vi "Parse JSON for Channels.vi"(8 "error in":errorcluster, 11 "JSON":string) -> (0 "error out":errorcluster, 2 "Channel JSON List":string[](array[string]), 3 "Channel Type List":string[](array[string]))   [LabVIEW 2026, in "Template Deployment Hooks.lvlib"]
uses:
  Template Deployment Hooks.lvlib
  <vilib>/regexp/Match Regular Expression.xnode
  <vilib>/JDP Science/JSONtext/JSONtext.lvlib
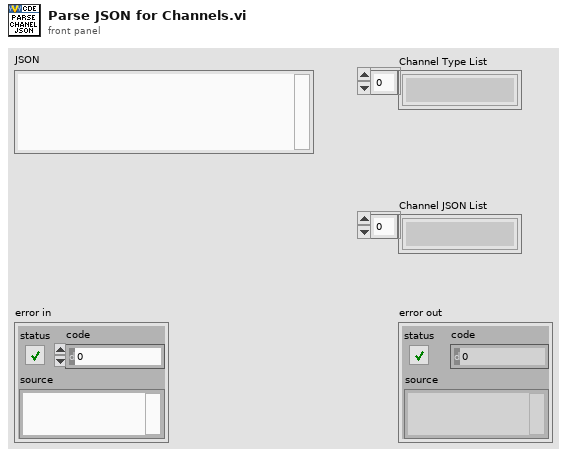
[diagram p1: front panel]
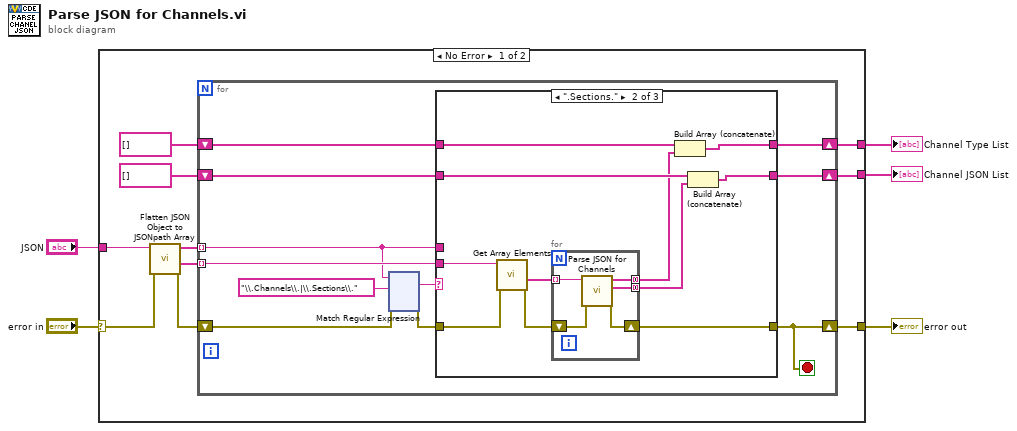
[diagram p0: block diagram]
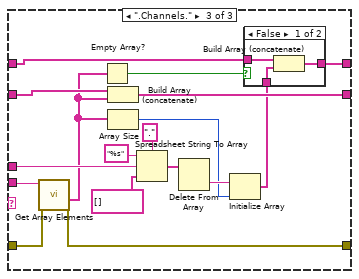
[diagram p3: hidden frame]
diagram:
  n1 = case shown="No Error" "error in" {
    selector: "error in" -> [w14 w184]
    tunnel: [w13 w184] -> w5
    tunnel: "JSON" -> [w9 _]
    tunnel: [w7 _] -> w2
    tunnel: [w6 _] -> w1
    frame No Error {
      n2 = call <vilib>:"Flatten JSON Object to JSONpath Array.vi"("error in (no error)"=w14, "JSON"=w9) -> ("error out"=w15:errorcluster, "<JSON>"=w11:string[], "$Paths"=w12:string[])  [unwired: 7 in]
      n3 = for {
        tunnel: w12 -> [w18] mode=indexing
        shift-right: [w22] -> w6
        shift-left: string[] [] ("<JSON>") -> [w23]
        tunnel: w11 -> [w21] mode=indexing
        shift-right: [w26] -> w13
        shift-left: w15 -> [w25]
        shift-right: [w19] -> w7
        shift-left: string[] [] -> [w20]
        stop <- w26 stop-if-true
        n4 = xnode "Match Regular Expression"("input string"=w18, "regular expression"="\\.Channels\\.|\\.Sections\\.", "error in"=w25) -> ("whole match"=w16:string, "error out"=w24:errorcluster)  [unwired: 3 in, 3 out]
        n5 = case shown="\".Sections.\"" w16 {
          tunnel: [w29 w38 w61] -> w26
          tunnel: w23 -> [w27 w37 w60]
          tunnel: [w27 w31 w59] -> w22
          tunnel: w21 -> [_ w36 w51]
          tunnel: w20 -> [w28 w35 w52]
          tunnel: [w28 w33 w53] -> w19
          tunnel: w24 -> [w29 w40 w62]
          tunnel: w18 -> [_ _ w54]
          frame Default {
          }
          frame ".Sections." {
            n6 = call <vilib>:"Get Array Elements.vi"("error in (no error)"=w40, "JSON"=w36) -> ("error out"=w39:errorcluster, "<JSON>"=w34:string[])  [unwired: 7 in, 1 out]
            n7 = for {
              tunnel: w34 -> [w43] mode=indexing
              tunnel: [w42] -> w32 mode=concatenating
              tunnel: [w41] -> w30 mode=concatenating
              shift-right: [w44] -> w38
              shift-left: w39 -> [w45]
              n8 = call "Parse JSON for Channels.vi"("error in"=w45, "JSON"=w43) -> ("error out"=w44:errorcluster, "Channel JSON List"=w41:string[], "Channel Type List"=w42:string[])  [unwired: 7 in]
            }
            n9 = Build Array (concatenate)(w35, w32) -> (w33:string[])
            n10 = Build Array (concatenate)(w37, w30) -> (w31:string[])
          }
          frame ".Channels." {
            n11 = call <vilib>:"Get Array Elements.vi"("error in (no error)"=w62, "JSON"=w51) -> ("error out"=w61:errorcluster, "<JSON>"=w49:string[])  [unwired: 7 in, 1 out]
            n12 = Empty Array?(array=w49) -> (empty?=w50:bool)
            n13 = Build Array (concatenate)(w60, w49) -> (w59:string[])
            n14 = Array Size(array=w49) -> (size(s)=w47:i32)
            n15 = Spreadsheet String To Array(delimiter (Tab)=".", format string="%s", spreadsheet string=w54, array type (2D Dbl)=string[] []) -> (array=w55:string[])
            n16 = Delete From Array(array=w55) -> (deleted portion=w48:string)  [unwired: 2 in, 1 out]
            n17 = Initialize Array(w48, w47) -> (w46:string[])
            n18 = case shown="False" w50 {
              tunnel: w46 -> [w65 _]
              tunnel: [w64 w66] -> w53
              tunnel: w52 -> [w63 w66]
              frame False {
                n19 = Build Array (concatenate)(w63, w65) -> (w64:string[])
              }
              frame True {
              }
            }
          }
        }
      }
    }
    frame Error {
    }
  }
  "error out" <- w5
  "Channel Type List" <- w2
  "Channel JSON List" <- w1
